vi "myCommOpen_visa.vi"(7 "log输入":string, 8 "错误输入（无错误）":errorcluster, 11 "与DSP连接的串口":refnum<visa-resource-name>) -> (0 "错误输出":errorcluster, 2 "是否有可用DSP":bool, 3 "VISA resource name out":refnum<visa-resource-name>, 5 "log输出":string)   [LabVIEW 2024]
uses:
  <vilib>/Instr/_visa.llb/VISA Configure Serial Port (Instr).vi
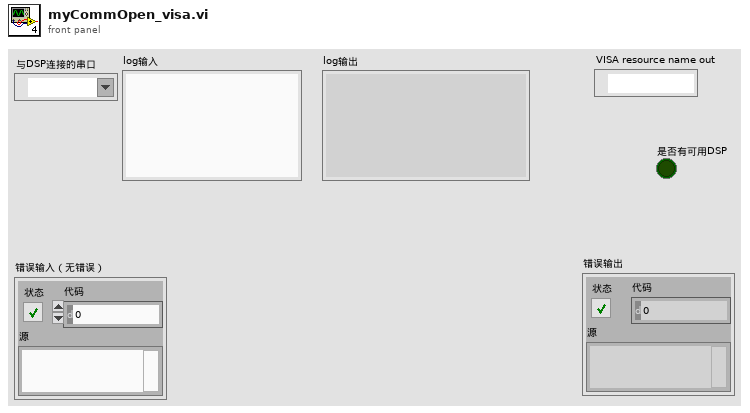
[diagram p1: front panel]
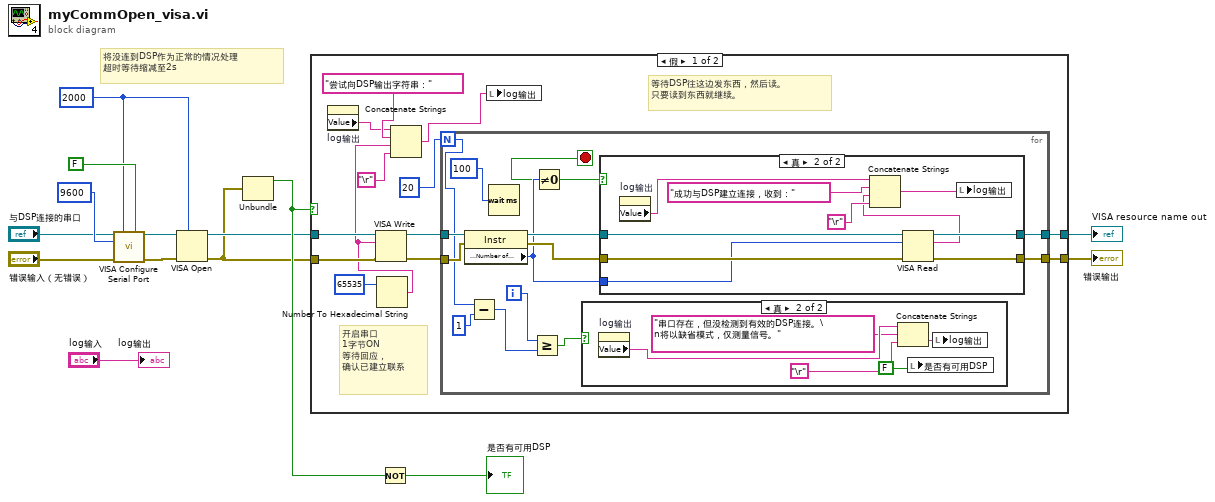
[diagram p0: block diagram]
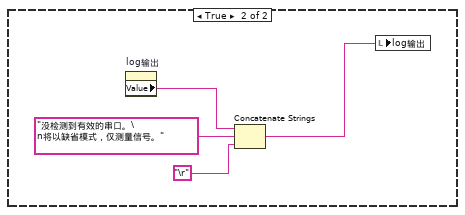
[diagram p4: hidden frame]
diagram:
  w4 = u32 2000 ("timeout (10sec)")
  # "将没连到DSP作为正常的情况处理\n超时等待缩减至2s"
  n1 = call-poly "VISA Configure Serial Port"("VISA resource name"="与DSP连接的串口", "timeout (10sec)"=w4, "Enable Termination\nChar (T)"=FALSE ("Enable Termination\nChar (T)"), "baud rate (9600)"=u32 9600 ("baud rate"), "error in (no error)"="错误输入（无错误）") -> ("VISA resource name out"=w6:refnum<visa-resource-name>, "error out"=w2:errorcluster)  [unwired: 9 in]
  n2 = VISA Open(timeout (0)=w4, error in (no error)=w2, VISA resource name=w6) -> (VISA resource name=w5:refnum<visa-resource-name>, error out=w3:errorcluster)  [unwired: 2 in]
  n3 = Unbundle(w3) -> ("status"=w8:bool)  [unwired: 2 out]
  n4 = case shown="假" w8 {
    tunnel: w5 -> [w27 _]
    tunnel: [w24 _] -> w10
    tunnel: [w23 _] -> w9
    tunnel: w3 -> [w22 _]
    frame False {
      # "开启串口\n1字节ON\n等待回应，\n确认已建立联系"
      # "等待DSP往这边发东西，然后读。\n只要读到东西就继续。"
      n5 = property on="log输出" class="Str"() -> ("Value"=w15:string)  [unwired: 2 in, 2 out]
      n6 = Number To Hexadecimal String(2:u16 65535) -> (0:w20:string)  [unwired: 1 in]
      n7 = VISA Write(VISA resource name=w27, write buffer=w20, error in (no error)=w22) -> (VISA resource name out=w26:refnum<visa-resource-name>, error out=w18:errorcluster)  [unwired: 1 out]
      n8 = Concatenate Strings(w15, "尝试向DSP输出字符串：", w20, "\r") -> (w17:string)
      n9 = for {
        N: 20 ("数值") -> [w31]
        tunnel: w26 -> [w41]
        tunnel: w18 -> [w40]
        tunnel: [w36] -> w23
        tunnel: [w35] -> w24
        i -> [w29]
        stop <- w33 stop-if-true
        n10 = property class="Instr"(reference=w41, error in=w40) -> (reference out=w39:refnum<visa-resource-name>, error out=w38:errorcluster, "Serial Settings:Number of Bytes at Serial Port"=w37:u32)
        n11 = Subtract(x=w31, y=1) -> (x-y=w30:i32)
        n12 = Wait (ms)(milliseconds to wait=u32 100 ("等待时间（毫秒）")) -> ()  [unwired: 1 out]
        n13 = Greater Or Equal?(x=w29, y=w30) -> (x >= y?=w28:bool)
        n14 = Not Equal To 0?(x=w37) -> (x != 0?=w33:bool)
        n15 = case shown="真" w28 {
          frame False {
          }
          frame True {
            n16 = property on="log输出" class="Str"() -> ("Value"=w46:string)  [unwired: 2 in, 2 out]
            n17 = Concatenate Strings(w46, "串口存在，但没检测到有效的DSP连接。\n将以缺省模式，仅测量信号。", "\r") -> (w43:string)
            n18 = local write "是否有可用DSP"(FALSE) -> ()
            n19 = local write "log输出"(w43) -> ()
          }
        }
        n20 = case shown="真" w33 {
          tunnel: w39 -> [w48 w57]
          tunnel: w38 -> [w47 w58]
          tunnel: w37 -> [_ w56]
          tunnel: [w47 w55] -> w36
          tunnel: [w48 w54] -> w35
          frame False {
          }
          frame True {
            n21 = property on="log输出" class="Str"() -> ("Value"=w51:string)  [unwired: 2 in, 2 out]
            n22 = VISA Read(VISA resource name=w57, byte count=w56, error in (no error)=w58) -> (VISA resource name out=w54:refnum<visa-resource-name>, read buffer=w50:string, error out=w55:errorcluster)  [unwired: 1 out]
            n23 = Concatenate Strings(w51, "成功与DSP建立连接，收到：", w50, "\r") -> (w49:string)
            n24 = local write "log输出"(w49) -> ()
          }
        }
      }
      n25 = local write "log输出"(w17) -> ()
    }
    frame True {
      n26 = property on="log输出" class="Str"() -> ("Value"=w59:string)  [unwired: 2 in, 2 out]
      n27 = Concatenate Strings(w59, "没检测到有效的串口。\n将以缺省模式，仅测量信号。", "\r") -> (w60:string)
      n28 = local write "log输出"(w60) -> ()
    }
  }
  "错误输出" <- w9
  "VISA resource name out" <- w10
  n29 = Not(x=w8) -> (.not. x?=→"是否有可用DSP":bool)
  "log输出" <- "log输入"
